vi "cv_08_03.vi"() -> ()   [LabVIEW 2013]
uses:
  <vilib>/regexp/Match Regular Expression.xnode
panel:
  out "error out":errorcluster
  out "Meter":dbl(knob) scale=0.0..24.0
  out "String":string
  in  "Unit to Write":string
  in  "Numeric to Write":dbl
  out "Path":path
  in  "String to Write":string
  out "Array":dbl[](array[numeric])
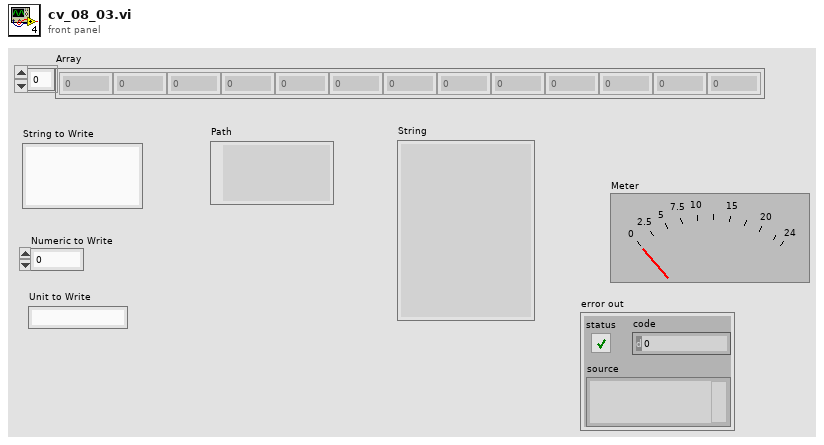
[diagram p1: front panel]
types:
  T1 = enum16{"open", "replace", "create", "open or create", "replace or create"}
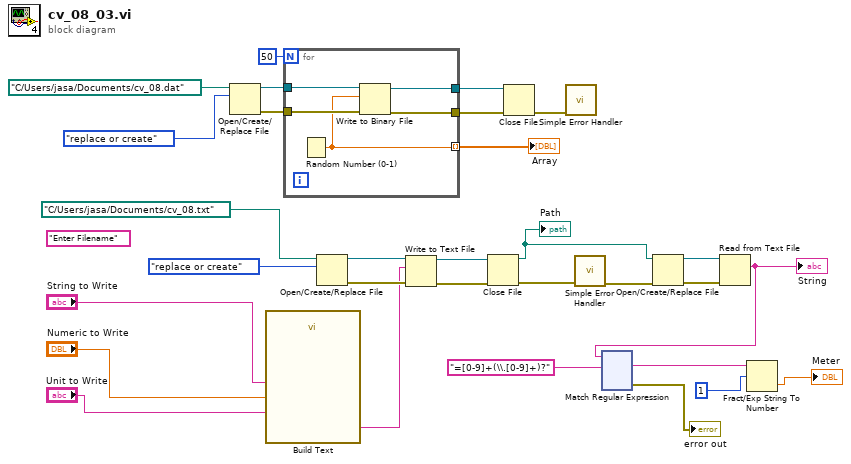
[diagram p0: block diagram]
diagram:
  (unwired) "Enter Filename"
  n1 = Open/Create/Replace File(file path (use dialog)=path "C:/Users/jasa/Documents/cv_08.dat", operation (0:open)=T1."replace or create") -> (refnum out=w28:refnum<file>, error out=w27:errorcluster)  [unwired: 4 in, 1 out]
  n2 = call "Build Text"("S1"="String to Write", "F1"="Numeric to Write", "S2"="Unit to Write") -> ("Result"=w13:string)  [unwired: 11 in, 1 out]
  n3 = for {
    N: 50 -> [_]
    tunnel: w28 -> [w35]
    tunnel: w27 -> [w34]
    tunnel: [w33] -> w26
    tunnel: [w32] -> w25
    tunnel: [w31] -> w22 mode=indexing
    n4 = Random Number (0-1)() -> (number: 0 to 1=w31:dbl)
    n5 = Write to Binary File(file (use dialog)=w35, data=w31, error in=w34) -> (refnum out=w33:refnum<file>, error out=w32:errorcluster)  [unwired: 3 in, 1 out]
  }
  "Array" <- w22
  n6 = Open/Create/Replace File(file path (use dialog)=path "C:/Users/jasa/Documents/cv_08.txt", operation (0:open)=T1."replace or create") -> (refnum out=w12:refnum<file>, error out=w20:errorcluster)  [unwired: 4 in, 1 out]
  n7 = Write to Text File(file (use dialog)=w12, text=w13, error in=w20) -> (refnum out=w19:refnum<file>, error out=w18:errorcluster)  [unwired: 1 in, 1 out]
  n8 = Close File(refnum=w19, error in=w18) -> (path=w10:path, error out=w17:errorcluster)
  "Path" <- w10
  n9 = Close File(refnum=w26, error in=w25) -> (error out=w24:errorcluster)  [unwired: 1 out]
  n10 = call <vilib>:"Simple Error Handler.vi"("error in (no error)"=w24) -> ()  [unwired: 4 in, 5 out]
  n11 = call <vilib>:"Simple Error Handler.vi"("error in (no error)"=w17) -> ("error out"=w11:errorcluster)  [unwired: 4 in, 4 out]
  n12 = Open/Create/Replace File(file path (use dialog)=w10, error in=w11) -> (refnum out=w8:refnum<file>, error out=w9:errorcluster)  [unwired: 4 in, 1 out]
  n13 = Read from Text File(file (use dialog)=w8, error in=w9) -> (text=w6:string)  [unwired: 2 in, 3 out]
  "String" <- w6
  n14 = xnode "Match Regular Expression"("input string"=w6, "regular expression"="=[0-9]+(\\.[0-9]+)?") -> ("whole match"=w3:string, "error out"=→"error out":errorcluster)  [unwired: 4 in, 3 out]
  n15 = Fract/Exp String To Number(string=w3, offset=1) -> (number=→"Meter":dbl)  [unwired: 2 in, 1 out]
